vi "Lockin-4461 IV mode trigger and wait.vi"(8 "error in (no error)":errorcluster, 11 "Channels: AO":T1={"AO amp (V)"=[1.0, 0.0, 0.0, 0.0, 0.0, 0.0, 0.0, 0.0], "AO DC (V)"=[0.0, 0.0, 0.0, 0.0, 0.0, 0.0, 0.0, 0.0], "AO f (Hz)"=[1.0, 1.0, 1.0, 1.0, 1.0, 1.0, 1.0, 1.0], "AO phi (deg)"=[0.0, 0.0, 0.0, 0.0, 0.0, 0.0, 0.0, 0.0], "function"=[enum."Triangle Wave", enum."Sine Wave", enum."Sine Wave", enum."Sine Wave", enum."Sine Wave", enum."Sine Wave", enum."Sine Wave", enum."Sine Wave"]} {"AO DC (V)" format="%#_6p"; "AO amp (V)" format="%#_6p"}) -> (0 "error out":errorcluster)   [LabVIEW 2013]
panel:
  in  "y":bool
  out "timer (s)":dbl=1.2239999771118164
  # "This VI triggers the lockin and waits until the acquisition is complete"
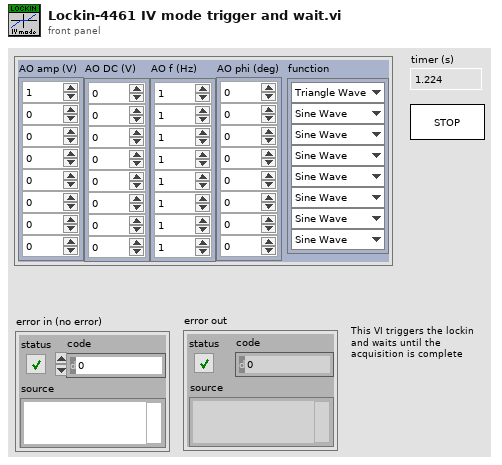
[diagram p1: front panel]
types:
  T1 = cluster{"AO amp (V)":dbl[], "AO DC (V)":dbl[], "AO f (Hz)":dbl[], "AO phi (deg)":dbl[], "function":enum16{"Sine Wave", "Triangle Wave", "Square Wave", "Sawtooth Wave"}[]}
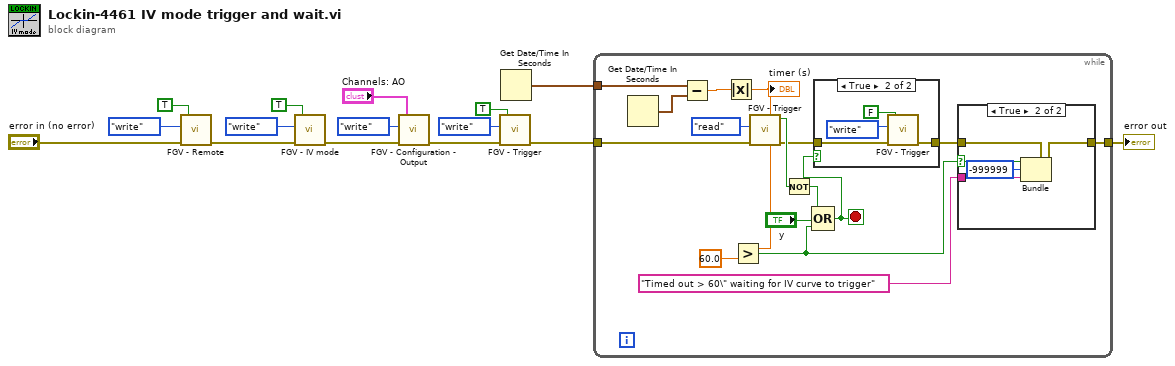
[diagram p0: block diagram]
diagram:
  n1 = call "FGV - Remote.vi"("error in"="error in (no error)", "Function"=enum16{"write", "read"}."write", "Remote Mode"=TRUE ("Trigger")) -> ("error out"=w7:errorcluster)  [unwired: 3 in, 1 out]
  n2 = call "FGV - IV mode.vi"("error in"=w7, "Function"=enum16{"write", "read"}."write", "IV mode"=TRUE ("Trigger")) -> ("error out"=w4:errorcluster)  [unwired: 3 in, 1 out]
  n3 = call "FGV - Configuration - Output.vi"("error in"=w4, "Function"=enum16{"write", "read"}."write", "Channels: AO"="Channels: AO") -> ("error out"=w3:errorcluster)  [unwired: 3 in, 1 out]
  n4 = call "FGV - Trigger.vi"("error in"=w3, "Function"=enum16{"write", "read"}."write", "Trigger"=TRUE) -> ("error out"=w13:errorcluster)  [unwired: 3 in, 1 out]
  n5 = Get Date/Time In Seconds() -> (seconds since 1Jan1904=w12:timestamp)
  n6 = while {
    tunnel: w13 -> [w27]
    tunnel: w12 -> [w30]
    tunnel: [w22] -> w11
    stop <- w16 stop-if-true
    n7 = Get Date/Time In Seconds() -> (seconds since 1Jan1904=w29:timestamp)
    n8 = Subtract(x=w30, y=w29) -> (x-y=w28:dbl)
    n9 = Absolute Value(x=w28) -> (abs(x)=w24:dbl)
    "timer (s)" <- w24
    n10 = Greater?(x=w24, y=60.0) -> (0:w17:bool)
    n11 = call "FGV - Trigger.vi"("error in"=w27, "Function"=enum16{"write", "read"}."read") -> ("error out"=w20:errorcluster, "Trigger 2"=w21:bool)  [unwired: 4 in]
    n12 = Not(x=w21) -> (.not. x?=w26:bool)
    n13 = Compound Arithmetic op=OR(w26, "y", w17) -> (w16:bool)
    n14 = case shown="True" w16 {
      tunnel: w20 -> [w32 w34]
      tunnel: [w32 w33] -> w19
      frame False {
      }
      frame True {
        n15 = call "FGV - Trigger.vi"("error in"=w34, "Function"=enum16{"write", "read"}."write", "Trigger"=FALSE) -> ("error out"=w33:errorcluster)  [unwired: 3 in, 1 out]
      }
    }
    n16 = case shown="True" w17 {
      selector: w17 -> [_ w40]
      tunnel: "Timed out > 60\" waiting for IV curve to trigger" ("source") -> [_ w42]
      tunnel: w19 -> [w37 w41]
      tunnel: [w37 w39] -> w22
      frame False {
      }
      frame True {
        n17 = Bundle(cluster=w41, "status"=w40, "code"=-999999, "source"=w42) -> (w39:errorcluster)
      }
    }
  }
  "error out" <- w11
